vi "Read TCP Reference.vi"(8 "error in (no error)":errorcluster, 11 "Vessel in":refnum<class "Vessel.lvclass">) -> (0 "error out":errorcluster, 2 "FPGA VI Reference Out":refnum<k20>, 3 "Vessel out":refnum<class "Vessel.lvclass">)   [LabVIEW 2012]
uses:
  Vessel.lvclass
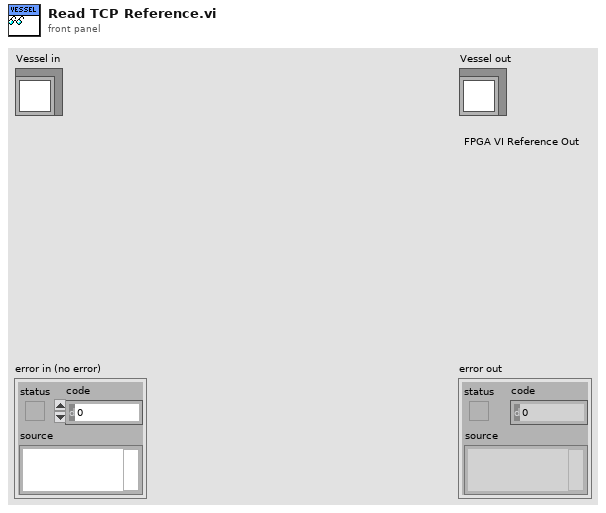
[diagram p1: front panel]
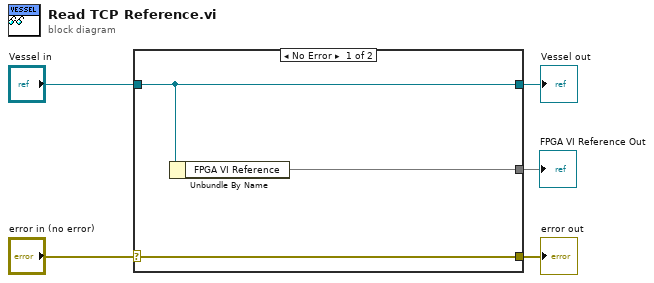
[diagram p0: block diagram]
diagram:
  n1 = case shown="No Error" "error in (no error)" {
    selector: "error in (no error)" -> [w8 w9]
    tunnel: [w8 w9] -> w4
    tunnel: [w7 w10] -> w2
    tunnel: "Vessel in" -> [w7 w10]
    tunnel: [w6 _] -> w1
    frame No Error {
      n2 = Unbundle By Name(w7) -> ("FPGA VI Reference"=w6)
    }
    frame Error {
    }
  }
  "error out" <- w4
  "Vessel out" <- w2
  "FPGA VI Reference Out" <- w1
